vi "Register Memory Event.vi"(8 "Error In":errorcluster, 10 "User Event":T1, 11 "Memory Object":T2 {"Dimension"."Width" min=1; "Dimension"."Height" min=1; "Dimension"."Depth" min=1}) -> (0 "Error Out":errorcluster, 2 "User Event Out":T1, 3 "Memory Object Out":T2 {"Dimension"."Width" min=1; "Dimension"."Height" min=1; "Dimension"."Depth" min=1})   [LabVIEW 2012, in "OpenCLV x64.lvlib"]
doc: "Registers a memory user event using a Boolean Labview User Event. Once memory has been registered with a Labview User Event, it can be read and written to asynchronously (non-blocking) to allow other tasks to be performed by the program including user inputs to the front panel.\n\nThis is useful when copying very large datasets to the device."
uses:
  OpenCLV x64.lvlib
  Controls/Memory Object.ctl
  Controls/Device ID.ctl
  Controls/Memory ID.ctl
  User Controls/Array Dimensions.ctl
  Controls/Memory Type.ctl
  Controls/User Event.ctl
  Error Checking/Add Error Functional Global.vi
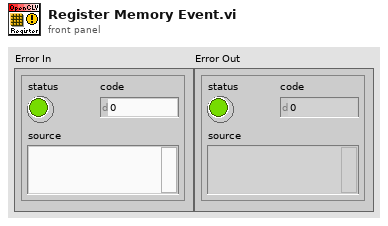
[diagram p1: front panel]
types:
  T1 = typedef "OpenCLV x64.lvlib/User Event.ctl" = refnum<user-event>
  T2 = typedef "OpenCLV x64.lvlib/Memory Object.ctl" = cluster{"Device ID":T3, "Memeroy ID":T4, "Dimension":T5, "Memory Type":T6}
  T3 = typedef "OpenCLV x64.lvlib/Device ID.ctl" = u64
  T4 = typedef "OpenCLV x64.lvlib/Memory ID.ctl" = u64
  T5 = typedef "Array Dimensions.ctl" = cluster{"Depth":u64, "Height":u64, "Width":u64}
  T6 = typedef "OpenCLV x64.lvlib/Memory Type.ctl" = enum16{"32f", "u8", "i8", "u16", "i16", "u32", "i32", "64f"}
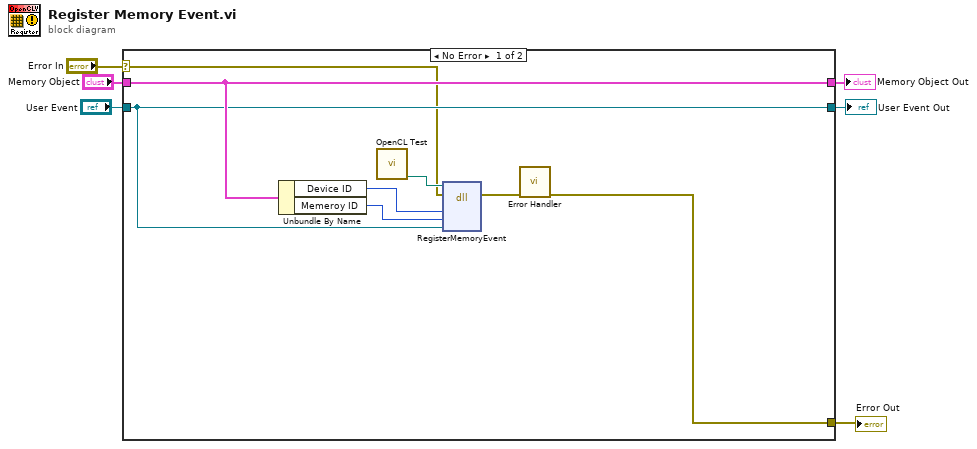
[diagram p0: block diagram]
diagram:
  n1 = case shown="No Error" "Error In" {
    selector: "Error In" -> [w7 w17]
    tunnel: [w8 w17] -> w5
    tunnel: "Memory Object" -> [w11 w15]
    tunnel: "User Event" -> [w10 w16]
    tunnel: [w11 w15] -> w3
    tunnel: [w10 w16] -> w1
    frame No Error {
      n2 = Unbundle By Name(w11) -> ("Device ID"=w12:T3, "Memeroy ID"=w13:T4)
      n3 = call "OpenCL Test.vi"() -> ("DLL To Use"=w14:path)  [unwired: 11 in]
      n4 = dll-call lib="D:/OpenCLV/trunk/OpenCLV_x64_1.0/OpenCLV_x64.dll" fn="RegisterMemoryEvent"(path in=w14, error in=w7, "Device"=w12, "Memory"=w13, "Labview Event"=w10) -> (error out=w9:errorcluster)  [unwired: 5 in, 1 out]
      n5 = call-poly "Error Handler.vi"("Error In"=w9) -> ("Error Out"=w8:errorcluster)  [unwired: 10 in]
    }
    frame Error {
    }
  }
  "Error Out" <- w5
  "Memory Object Out" <- w3
  "User Event Out" <- w1
